vi "Get or Add Style Index by Format.vi"(8 "error in":errorcluster, 10 "Format":string="dd/mm/yy hh:mm:ss.000", 11 "SpreadsheetDoc in":refnum<k24>) -> (0 "error out":errorcluster, 2 "Style Index":u32, 3 "SpreadsheetDoc out":refnum<k24>)   [LabVIEW 2021, in "Open Xml.lvlib"]
uses:
  Open Xml.lvlib
  D:/git/Open-Xml-LabVIEW/dll/DocumentFormat.OpenXml.dll
  dll/DocumentFormat.OpenXml.dll
  D:/git/Open-Xml-LabVIEW/dll/DocumentFormat.OpenXml.Framework.dll
  dll/DocumentFormat.OpenXml.Framework.dll
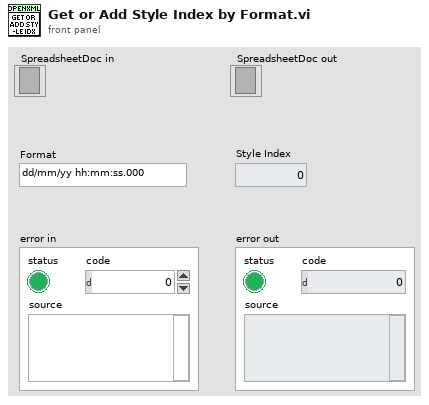
[diagram p1: front panel]
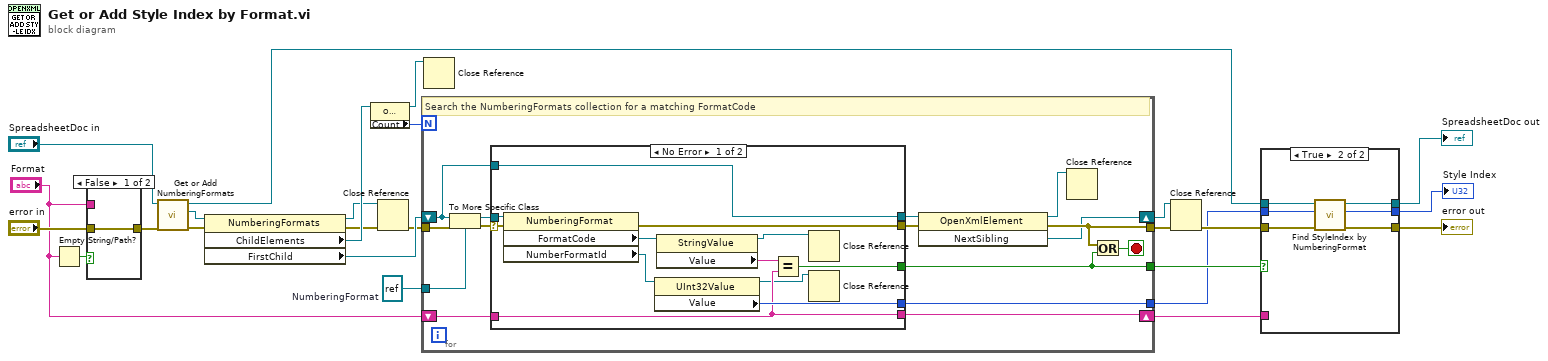
[diagram p0: block diagram]
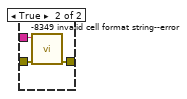
[diagram p2: hidden frame]
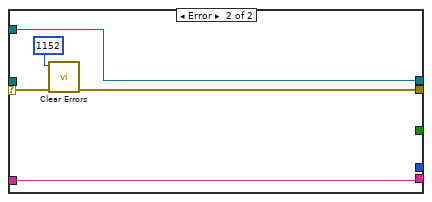
[diagram p3: hidden frame]
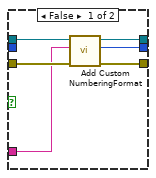
[diagram p4: hidden frame]
diagram:
  w20 = refnum<k24> refnum  # NumberingFormat
  n1 = Empty String/Path?(string/path="Format") -> (empty?=w17:bool)
  n2 = case shown="False" w17 {
    tunnel: "error in" -> [w26 w29]
    tunnel: [w26 w28] -> w18
    tunnel: "Format" -> [_ w27]
    frame False {
    }
    frame True {
      n3 = call "-8349 invalid cell format string--error.vi"("error in"=w29, "Argument"=w27) -> ("error out"=w28:errorcluster)  [unwired: 9 in]
    }
  }
  n4 = call "Get or Add NumberingFormats.vi"("error in"=w18, "SpreadsheetDoc in"="SpreadsheetDoc in") -> ("error out"=w24:errorcluster, "NumberingFormats"=w22:refnum<k24>, "SpreadsheetDoc out"=w3:refnum<k24>)  [unwired: 7 in]
  n5 = property class="NumberingFormats"(reference=w22, error in=w24) -> (reference out=w4:refnum<k24>, error out=w12:errorcluster, "ChildElements"=w21:refnum<k24>, "FirstChild"=w11:refnum<k24>)
  n6 = property class="OpenXmlElementList"(reference=w21) -> (reference out=w19:refnum<k24>, "Count"=w7:i32)  [unwired: 1 in, 1 out]
  n7 = Close Reference(reference=w4, error in (no error)=w12) -> (error out=w5:errorcluster)
  n8 = for {
    N: w7 -> [_]
    tunnel: w5 -> [w43]
    tunnel: w20 -> [w44]
    shift-right: [w34] -> w8
    shift-left: w11 -> [w30]
    tunnel: [w36] -> w14
    tunnel: [w37] -> w15
    tunnel: [w32] -> w1
    shift-right: [w31] -> w13
    shift-left: "Format" -> [w39]
    stop <- w38 stop-if-true
    # "Search the NumberingFormats collection for a matching FormatCode"
    n9 = To More Specific Class(target class=w44, reference=w30, error in=w43) -> (specific class reference=w40:refnum<k24>, error out=w42:errorcluster)
    n10 = case shown="No Error" w42 {
      selector: w42 -> [w56 w61]
      tunnel: [w55 w60] -> w41
      tunnel: w40 -> [w54 _]
      tunnel: w39 -> [w48 w57]
      tunnel: [w51 _] -> w37
      tunnel: [w47 w58] -> w35
      tunnel: [w49 _] -> w32
      tunnel: [w48 w57] -> w31
      tunnel: w30 -> [w47 w58]
      frame No Error {
        n11 = property class="NumberingFormat"(reference=w54, error in=w56) -> (error out=w55:errorcluster, "FormatCode"=w53:refnum<k24>, "NumberFormatId"=w50:refnum<k24>)  [unwired: 1 out]
        n12 = property class="UInt32Value"(reference=w50) -> (reference out=w45:refnum<k24>, "Value"=w49:u32)  [unwired: 1 in, 1 out]
        n13 = property class="StringValue"(reference=w53) -> (reference out=w46:refnum<k24>, "Value"=w52:string)  [unwired: 1 in, 1 out]
        n14 = Equal?(x=w52, y=w48) -> (x = y?=w51:bool)
        n15 = Close Reference(reference=w46) -> ()  [unwired: 1 in, 1 out]
        n16 = Close Reference(reference=w45) -> ()  [unwired: 1 in, 1 out]
      }
      frame Error {
        n17 = call <vilib>:"Clear Errors.vi"("error in (no error)"=w61, "specific error code to clear (0: all)"=1152) -> ("error out"=w60:errorcluster)  [unwired: 4 in, 1 out]
      }
    }
    n18 = invoke class="OpenXmlElement" method="NextSibling"(reference=w35, error in=w41) -> (reference out=w33:refnum<k24>, error out=w36:errorcluster, "NextSibling"=w34:refnum<k24>)  [unwired: 1 in]
    n19 = Close Reference(reference=w33) -> ()  [unwired: 1 in, 1 out]
    n20 = Or(x=w36, y=w37) -> (x .or. y?=w38:bool)
  }
  n21 = Close Reference(reference=w19) -> ()  [unwired: 1 in, 1 out]
  n22 = Close Reference(reference=w8, error in (no error)=w14) -> (error out=w2:errorcluster)
  n23 = case shown="True" w15 {
    tunnel: w13 -> [w62 _]
    tunnel: w3 -> [w67 w71]
    tunnel: [w66 w70] -> w10
    tunnel: [w65 w68] -> w9
    tunnel: w2 -> [w64 w73]
    tunnel: [w63 w72] -> w6
    tunnel: w1 -> [_ w69]
    frame False {
      n24 = call "Add Custom NumberingFormat.vi"("error in"=w64, "Format"=w62, "Spreadsheet Doc in"=w67) -> ("error out"=w63:errorcluster, "StyleIndex"=w65:u32, "SpreadsheetDoc out"=w66:refnum<k24>)  [unwired: 6 in]
    }
    frame True {
      n25 = call "Find StyleIndex by NumberingFormat.vi"("error in"=w73, "NumberingFormat Id"=w69, "Spreadsheet Doc in"=w71) -> ("error out"=w72:errorcluster, "StyleIndex"=w68:u32, "SpreadsheetDoc out"=w70:refnum<k24>)  [unwired: 6 in]
    }
  }
  "SpreadsheetDoc out" <- w10
  "error out" <- w6
  "Style Index" <- w9
